vi "ControlRoom-FPGA.vi"() -> ()   [LabVIEW 2016]
doc: "Fpga for Control room rio"
uses:
  Terminal Readback.ctl
  Chain Readbacks.ctl
  <vilib>/Platform/TimedLoop/XDataNode/timing_clust.ctl
  <vilib>/Platform/TimedLoop/XDataNode/nitl_modes.ctl
  <vilib>/Platform/TimedLoop/XDataNode/wakeup.ctl
  <vilib>/rvi/FXPMathLib/basic elements/FxpIntAccumulator/subVIs/nifxpmath_IntAccumulator_SimConfig.ctl
  <vilib>/rvi/Emulation/niFpgaGetClockAttributes.vi
  <vilib>/rvi/Emulation/niFpgaSctlEmulationGetInTimedLoop.vi
  <vilib>/rvi/Emulation/niFpgaEmulationReportErrorSimple.vi
  <vilib>/rvi/eio/common/nirviEmuTemplateMethod_errors.vi
  <vilib>/rvi/Analysis/common/codeGenErrors/XNode/niFpgaXNodeCodeGenErrorHandle.vi
  <vilib>/rvi/Emulation/niFpgaCriticalErrorInLSC.vi
  <vilib>/rvi/FXPMathLib/basic elements/FxpIntAccumulator/simVIs/DllFxpIntAccumulator_sub.vi
  <vilib>/eio/EIONode/EIONode.xnode
  <vilib>/rvi/Analysis/measure/dc-rms/XNode/niFpgaDC-RMS.xnode
  <vilib>/Platform/TimedLoop/XDataNode/XDataNode.xnode
  <vilib>/rvi/FXPMathLib/basic elements/FxpIntAccumulator/XNode/nifxpmath_IntAccumulator.xnode
  <vilib>/rvi/FXPMathLib/FxpMul/XNode/nifxpmath_Multiplier.xnode
  <vilib>/Platform/TimedLoop/XDataNode/XDNodeRunTimeDep.lvlib
  <vilib>/rvi/FXPMathLib/sim/FxpSim.dll
panel:
  in  "RT error":bool
  out "HE Readbacks":T1
  out "LE Readbacks":T1
  out "Terminal Readbacks":T2
  out "terminal voltage":fxp<+/-,26,5> format="%.23g"
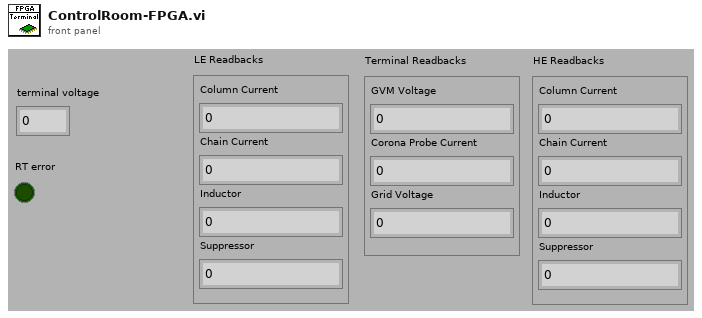
[diagram p1: front panel]
types:
  T1 = typedef "Chain Readbacks.ctl" = cluster{"Column Current":fxp<+/-,26,5>, "Chain Current":fxp<+/-,26,5>, "Inductor":fxp<+/-,26,5>, "Suppressor":fxp<+/-,26,5>}
  T2 = typedef "Terminal Readback.ctl" = cluster{"GVM Voltage ":fxp<+/-,26,5>, "Corona Probe Current":fxp<+/-,26,5>, "Grid Voltage":fxp<+/-,26,5>}
  T3 = typedef "XDNodeRunTimeDep.lvlib/timing_clust.ctl" = cluster{"Expected End [f-1]":u64, "Actual End [f-1]":u64, "Finished Late? [f-1]":bool, "Expected End [i-1]":u64, "Actual End [i-1]":u64, "Finished Late? [i-1]":bool, "Expected Start [i]":u64, "Actual Start [i]":u64, "Expected Start [f]":u64, "Actual Start [f]":u64, "Source Name":string, "Structure Name":string, "Period":i64, "Deadline":i64, "Offset":i64, "Start":i64, "Priority":i32, "Timeout":i32, "Mode":T4, "Wakeup Reason":T5, "Error":errorcluster, "Source Type":string, "Secondary Source Type":string, "Global End Time":u64, "Global Start Time":u64, "Frame Duration":u64, "Iteration Duration":u64, "Assigned CPU":i32, "I/O Scan Engine Mode":u32}
  T4 = typedef "XDNodeRunTimeDep.lvlib/nitl_modes.ctl" = enum32{"No Change", "Process missed periods, maintain original phase", "Discard missed periods, maintain original phase", "Process missed periods, ignore original phase", "Discard missed periods, ignore original phase"}
  T5 = typedef "XDNodeRunTimeDep.lvlib/wakeup.ctl" = enum32{"Normal", "Aborted", "Asynchronous wakeup", "Timing source error", "Timed loop error", "Timeout"}
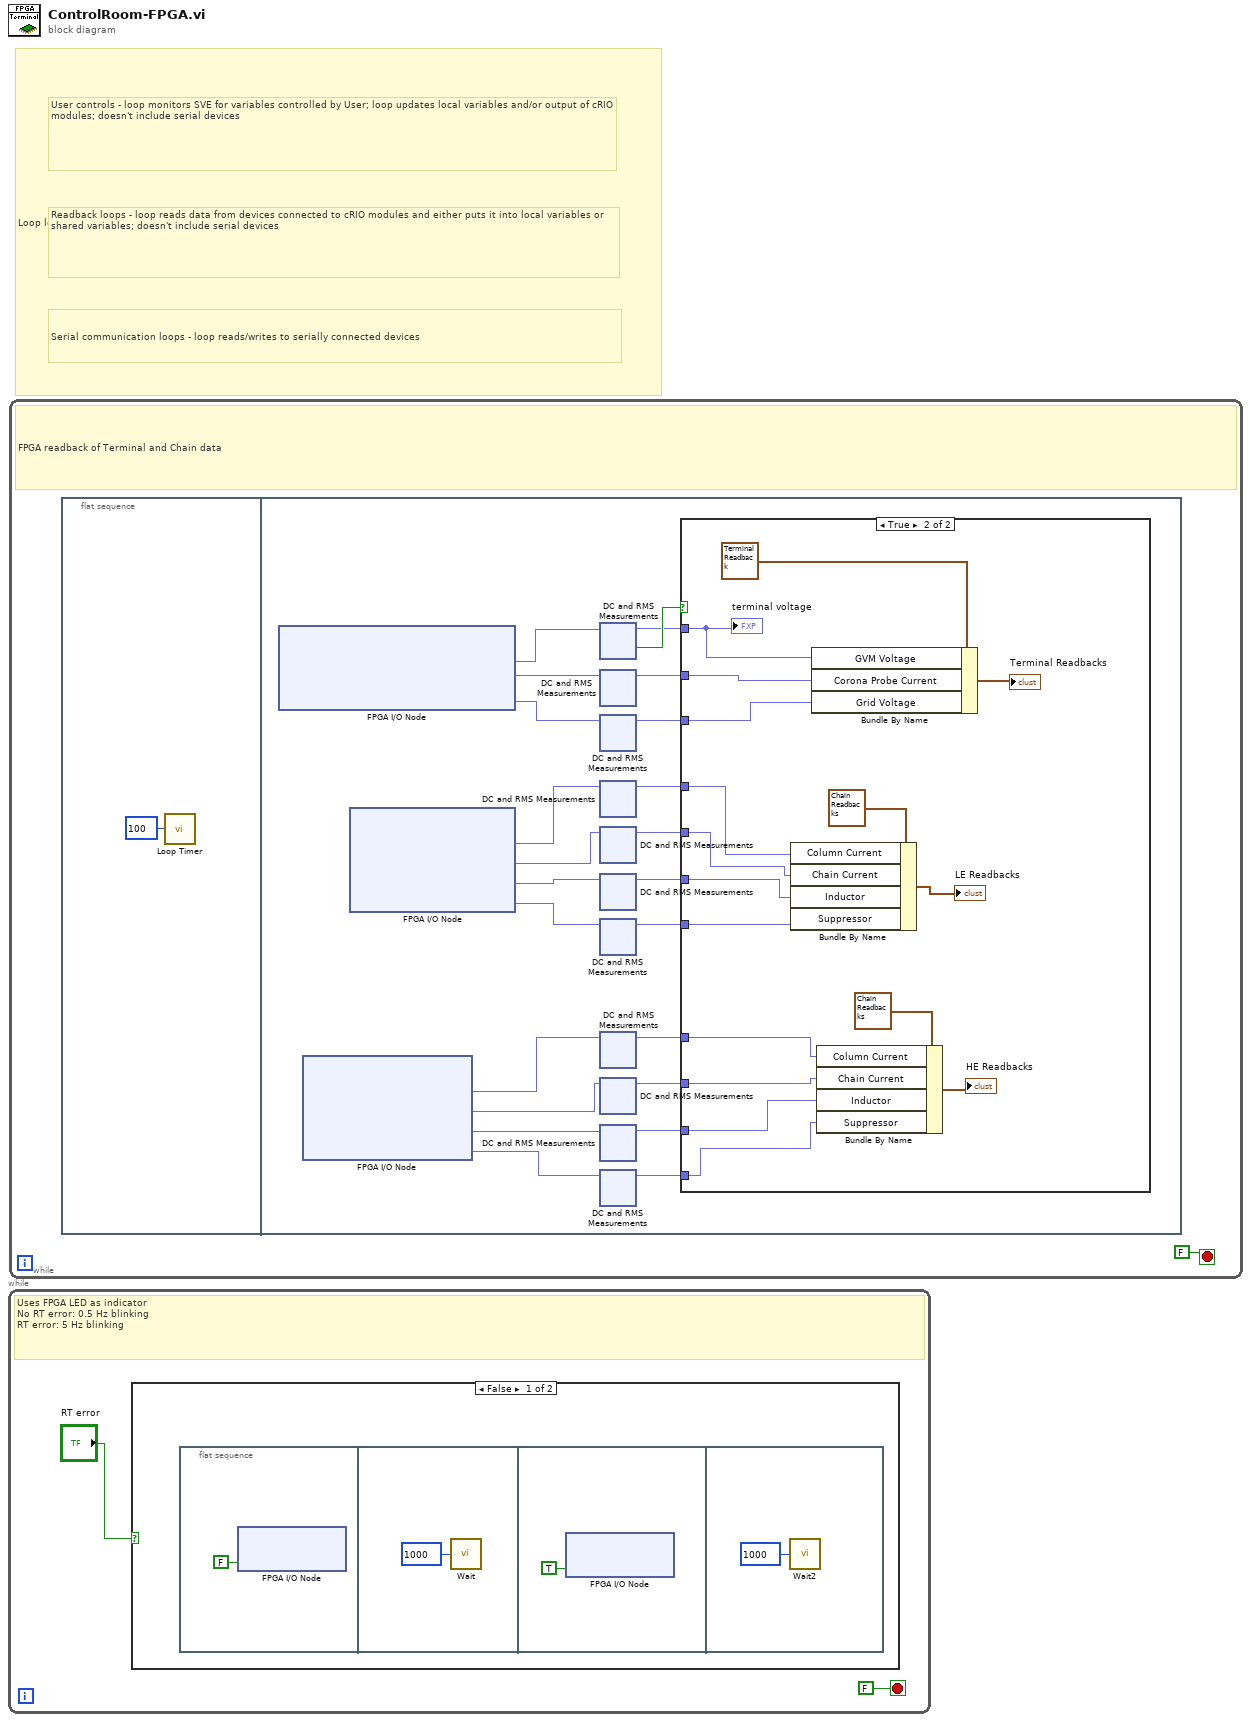
[diagram p0: block diagram]
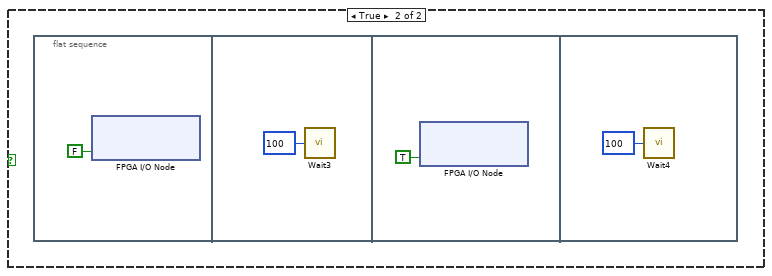
[diagram p2: hidden frame]
diagram:
  # "Serial communication loops - loop reads/writes to serially connected devices"
  # "Readback loops - loop reads data from devices connected to cRIO modules and either puts it into local variables or shared variables; doesn't include serial devices"
  # "User controls - loop monitors SVE for variables controlled by User; loop updates local variables and/or output of cRIO modules; doesn't include serial devices"
  # "Loop legend - loops are color coded by responsibility"
  n1 = while {
    stop <- FALSE stop-if-true
    # "Uses FPGA LED as indicator\nNo RT error: 0.5 Hz blinking\nRT error: 5 Hz blinking"
    n2 = case shown="False" "RT error" {
      frame False {
        n3 = flat-sequence {
          frame #0 {
            n4 = xnode "FPGA I/O Node"("FPGA LED"=FALSE) -> ()  [unwired: 1 in, 1 out]
          }
          frame #1 {
            n5 = call "Wait"("Count(mSec)"=u16 1000) -> ()  [unwired: 1 out]
          }
          frame #2 {
            n6 = xnode "FPGA I/O Node"("FPGA LED"=TRUE) -> ()  [unwired: 1 in, 1 out]
          }
          frame #3 {
            n7 = call "Wait2"("Count(mSec)"=u16 1000) -> ()  [unwired: 1 out]
          }
        }
      }
      frame True {
        n8 = flat-sequence {
          frame #0 {
            n9 = xnode "FPGA I/O Node"("FPGA LED"=FALSE) -> ()  [unwired: 1 in, 1 out]
          }
          frame #1 {
            n10 = call "Wait3"("Count(mSec)"=u16 100) -> ()  [unwired: 1 out]
          }
          frame #2 {
            n11 = xnode "FPGA I/O Node"("FPGA LED"=TRUE) -> ()  [unwired: 1 in, 1 out]
          }
          frame #3 {
            n12 = call "Wait4"("Count(mSec)"=u16 100) -> ()  [unwired: 1 out]
          }
        }
      }
    }
  }
  n13 = while {
    stop <- FALSE stop-if-true
    # "FPGA readback of Terminal and Chain data"
    n14 = flat-sequence {
      frame #0 {
        n15 = call "Loop Timer"("Count(uSec)"=u32 100 ("Count(Ticks)")) -> ()  [unwired: 1 out]
      }
      frame #1 {
        n16 = xnode "FPGA I/O Node"() -> ("GVM Voltage Output"=w35:fxp<+/-,26,5>, "Corona Probe Current Output"=w34:fxp<+/-,26,5>, "Grid Voltage Output"=w33:fxp<+/-,26,5>)  [unwired: 3 in, 3 out]
        n17 = xnode "FPGA I/O Node"() -> ("HE Column Current"=w28:fxp<+/-,26,5>, "HE Chain Current"=w27:fxp<+/-,26,5>, "HE Inductor"=w26:fxp<+/-,26,5>, "HE Suppressor"=w25:fxp<+/-,26,5>)  [unwired: 4 in, 4 out]
        n18 = xnode "FPGA I/O Node"() -> ("LE Column Current"=w32:fxp<+/-,26,5>, "LE Chain Current"=w31:fxp<+/-,26,5>, "LE Inductor"=w30:fxp<+/-,26,5>, "LE Suppressor"=w29:fxp<+/-,26,5>)  [unwired: 4 in, 4 out]
        n19 = xnode "DC and RMS Measurements"("input data"=w35) -> ("DC"=w23:fxp<+/-,26,5>, "output valid"=w24:bool)  [unwired: 1 in]
        n20 = xnode "DC and RMS Measurements"("input data"=w34) -> ("DC"=w22:fxp<+/-,26,5>)  [unwired: 1 in, 1 out]
        n21 = xnode "DC and RMS Measurements"("input data"=w33) -> ("DC"=w21:fxp<+/-,26,5>)  [unwired: 1 in, 1 out]
        n22 = xnode "DC and RMS Measurements"("input data"=w32) -> ("DC"=w20:fxp<+/-,26,5>)  [unwired: 1 in, 1 out]
        n23 = xnode "DC and RMS Measurements"("input data"=w31) -> ("DC"=w19:fxp<+/-,26,5>)  [unwired: 1 in, 1 out]
        n24 = xnode "DC and RMS Measurements"("input data"=w30) -> ("DC"=w18:fxp<+/-,26,5>)  [unwired: 1 in, 1 out]
        n25 = xnode "DC and RMS Measurements"("input data"=w29) -> ("DC"=w17:fxp<+/-,26,5>)  [unwired: 1 in, 1 out]
        n26 = xnode "DC and RMS Measurements"("input data"=w28) -> ("DC"=w16:fxp<+/-,26,5>)  [unwired: 1 in, 1 out]
        n27 = xnode "DC and RMS Measurements"("input data"=w27) -> ("DC"=w13:fxp<+/-,26,5>)  [unwired: 1 in, 1 out]
        n28 = xnode "DC and RMS Measurements"("input data"=w26) -> ("DC"=w15:fxp<+/-,26,5>)  [unwired: 1 in, 1 out]
        n29 = xnode "DC and RMS Measurements"("input data"=w25) -> ("DC"=w14:fxp<+/-,26,5>)  [unwired: 1 in, 1 out]
        n30 = case shown="True" w24 {
          tunnel: w23 -> [_ w916]
          tunnel: w22 -> [_ w929]
          tunnel: w21 -> [_ w932]
          tunnel: w20 -> [_ w926]
          tunnel: w19 -> [_ w925]
          tunnel: w18 -> [_ w924]
          tunnel: w17 -> [_ w923]
          tunnel: w16 -> [_ w920]
          tunnel: w15 -> [_ w918]
          tunnel: w14 -> [_ w917]
          tunnel: w13 -> [_ w919]
          frame False {
          }
          frame True {
            n31 = Bundle By Name(cluster=T1 {"Column Current"=0.0, "Chain Current"=0.0, "Inductor"=0.0, "Suppressor"=0.0} ("LE Readbacks 2"), "Column Current"=w926, "Chain Current"=w925, "Inductor"=w924, "Suppressor"=w923) -> (→"LE Readbacks":T1)
            n32 = Bundle By Name(cluster=T2 {"GVM Voltage "=0.0, "Corona Probe Current"=0.0, "Grid Voltage"=0.0} ("Terminal Readbacks 2"), "GVM Voltage"=w916, "Corona Probe Current"=w929, "Grid Voltage"=w932) -> (→"Terminal Readbacks":T2)
            n33 = Bundle By Name(cluster=T1 {"Column Current"=0.0, "Chain Current"=0.0, "Inductor"=0.0, "Suppressor"=0.0} ("LE Readbacks 2"), "Column Current"=w920, "Chain Current"=w919, "Inductor"=w918, "Suppressor"=w917) -> (→"HE Readbacks":T1)
            "terminal voltage" <- w916
          }
        }
      }
    }
  }
